vi "Get LakeShore 340 Data.vi"(8 "error in (no error)":errorcluster, 10 "Input (A or B)":string="A", 11 "VISA Resource Name":refnum<visa-resource-name>) -> (0 "error out":errorcluster, 1 "Raw":dbl, 2 "Temperature":dbl, 3 "VISA Resource Name Out":refnum<visa-resource-name>)   [LabVIEW 2015]
uses:
  GPIB/VISA  Send Receive.vi
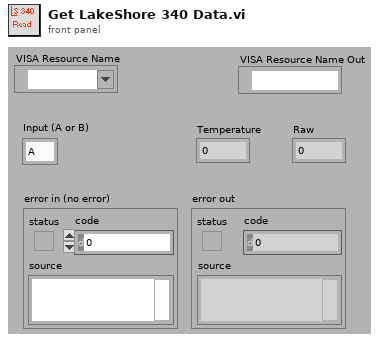
[diagram p1: front panel]
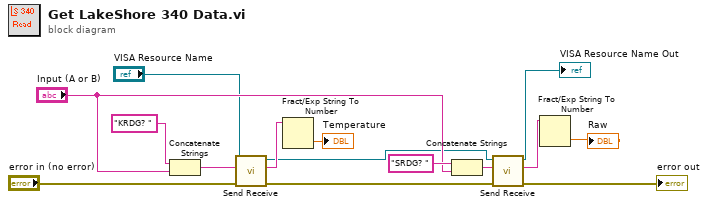
[diagram p0: block diagram]
diagram:
  n1 = Concatenate Strings("KRDG? " ("data string in"), "Input (A or B)") -> (w7:string)
  n2 = call-poly "Send Receive.vi"("error in (no error)"="error in (no error)", "data string in"=w7, "VISA Resource Name"="VISA Resource Name") -> ("error out"=w10:errorcluster, "data string out"=w14:string, "VISA Resource Name Out"=w2:refnum<visa-resource-name>)  [unwired: 6 in]
  n3 = Fract/Exp String To Number(string=w14) -> (number=→"Temperature":dbl)  [unwired: 4 out]
  n4 = Concatenate Strings("SRDG? " ("data string in"), "Input (A or B)") -> (w6:string)
  n5 = call-poly "Send Receive.vi"("error in (no error)"=w10, "data string in"=w6, "VISA Resource Name"=w2) -> ("error out"=→"error out":errorcluster, "data string out"=w12:string, "VISA Resource Name Out"=→"VISA Resource Name Out":refnum<visa-resource-name>)  [unwired: 6 in]
  n6 = Fract/Exp String To Number(string=w12) -> (number=→"Raw":dbl)  [unwired: 4 out]
